vi "Main Page.vi"(8 "error in (no error)":errorcluster, 11 "Node Ptr":T3 format="%.0x") -> (0 "error out":errorcluster)   [LabVIEW 2018, in "CAN Gateway System Explorer.lvlib"]
uses:
  CAN Gateway System Explorer.lvlib
  <vilib>/NI Veristand/Custom Device API/Custom Device Item Ref.ctl
  Types/Baudrate Network Port.ctl
  Types/Baudrate DUT Port.ctl
  Types/BR Cluster.ctl
  Shared/Constants.vi
  <vilib>/NI Veristand/Custom Device API/Get Item Property (String).vi
  <vilib>/NI Veristand/Custom Device API/Set Item Property (String).vi
  <vilib>/NI Veristand/Custom Device API/Set Item Property (Variant).vi
  <vilib>/NI Veristand/Custom Device API/Custom Device API.lvlib
  Shared/CAN Gateway Shared.lvlib
panel:
  in  "CLUSTER":u16(ring)
  in  "Baudrate DUT Port":T1 items=["1 M", "500k", "250 k", "125 k", "50k"]
  in  "Baudrate Network Port":T2 items=["1 M", "500k", "250 k", "125 k", "50k"]
  out "NETWORK --> DUT Frames":string[][](table)
  out "DUT --> NETWORK Frames":string[][](table)
  in  "DUT PORT":u16(ring)
  in  "ECU":u16(ring)
  in  "NETWORK PORT":u16(ring)
  out "Database Path":string
  in  "Header":cluster{"Section Name":string}={"Section Name"="CAN Gateway Custom Device"}
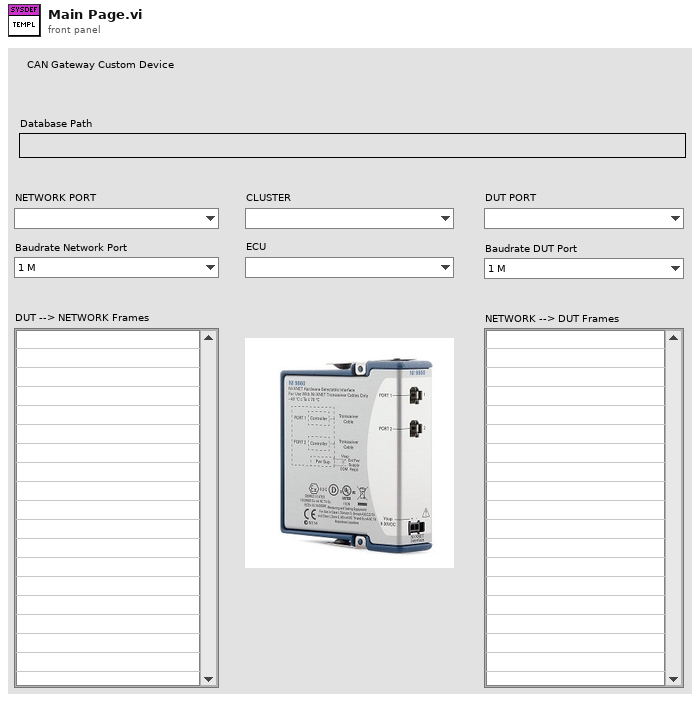
[diagram p1: front panel]
types:
  T1 = typedef "CAN Gateway System Explorer.lvlib/Baudrate DUT Port.ctl" = u16
  T2 = typedef "CAN Gateway System Explorer.lvlib/Baudrate Network Port.ctl" = u16
  T3 = typedef "Custom Device API.lvlib/Custom Device Item Ref.ctl" = u64
  T4 = typedef "CAN Gateway System Explorer.lvlib/BR Cluster.ctl" = cluster{"BR Network-Port":u16, "BR Port Network":u16}
  T5 = typedef "Custom Device API.lvlib/Custom Device Commands.ctl" = enum16{"Default", "Item renamed", "Shutdown", "Dynamic button pressed"}
  T6 = typedef "Custom Device API.lvlib/Custom Device Item Info.ctl" = cluster{"Name":string, "Is Channel":bool, "GUID":string, "Is Waveform":bool}
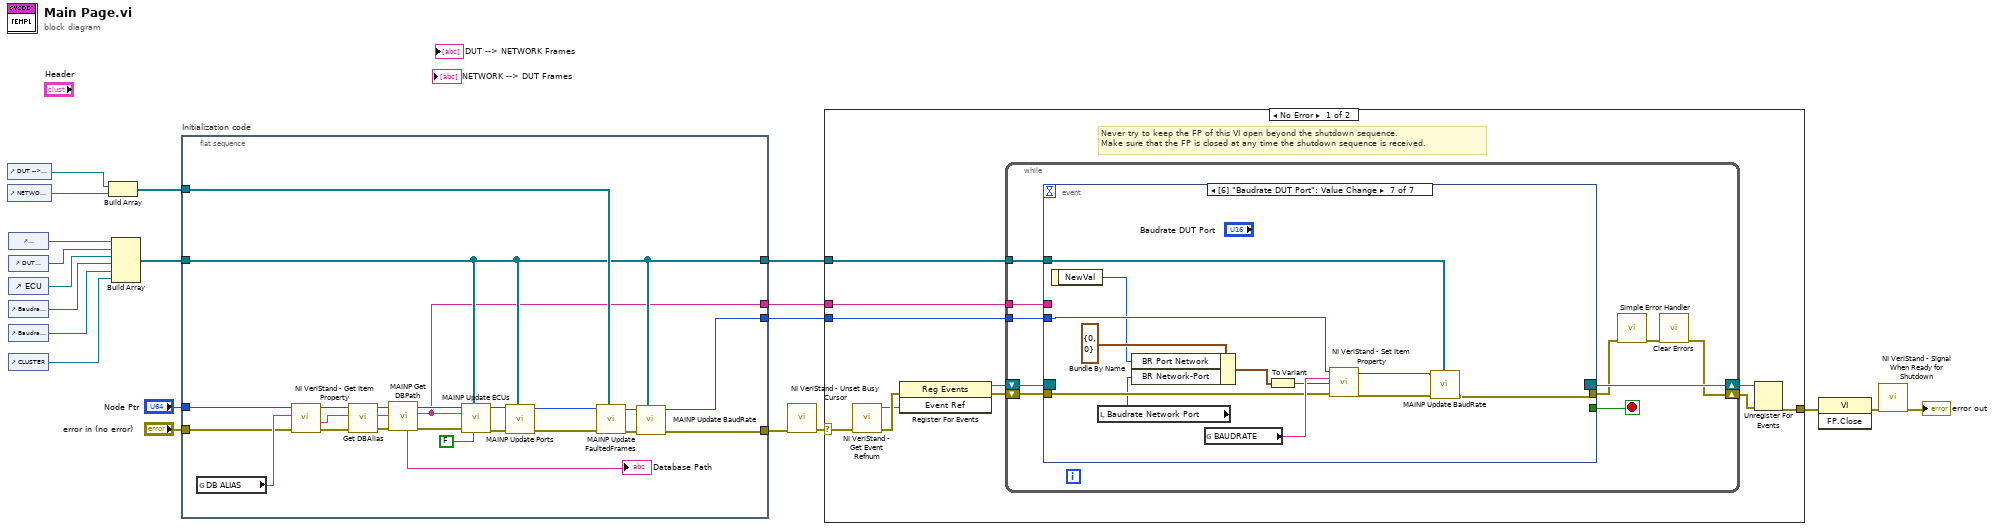
[diagram p0: block diagram]
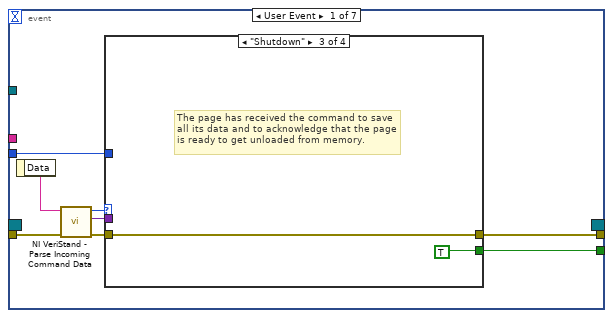
[diagram p2: hidden frame]
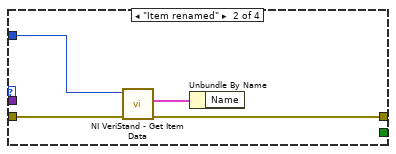
[diagram p4: hidden frame]
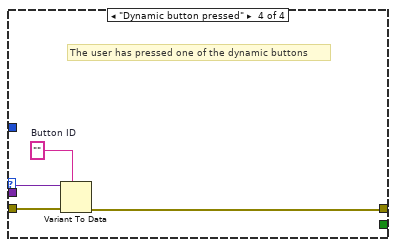
[diagram p5: hidden frame]
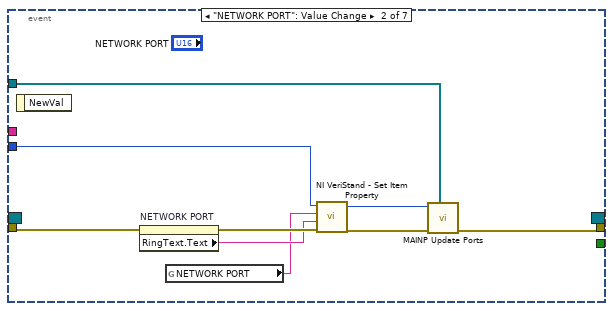
[diagram p6: hidden frame]
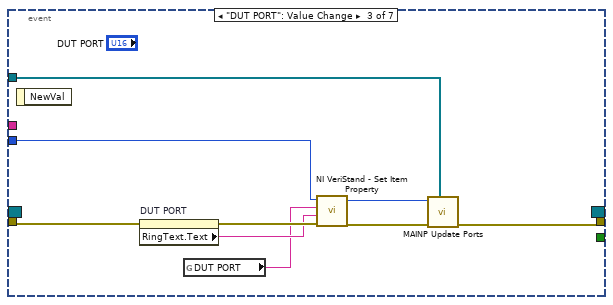
[diagram p7: hidden frame]
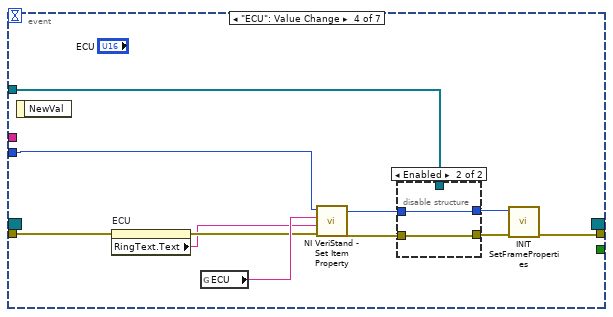
[diagram p8: hidden frame]
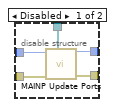
[diagram p9: hidden frame]
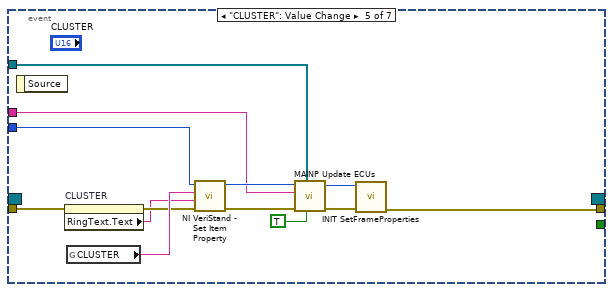
[diagram p10: hidden frame]
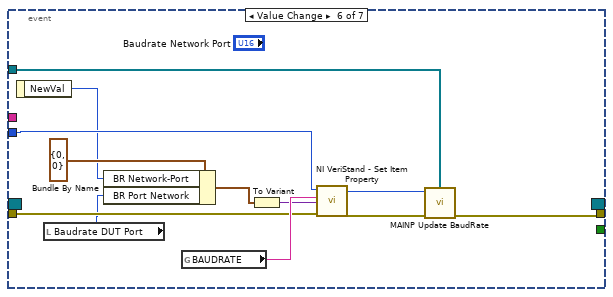
[diagram p11: hidden frame]
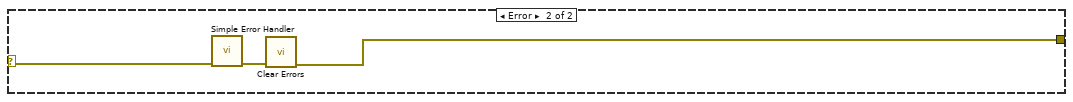
[diagram p12: hidden frame]
diagram:
  n1 = control-ref of="DUT --> NETWORK Frames"() -> (w6:refnum<vi>)
  n2 = control-ref of="NETWORK --> DUT Frames"() -> (w5:refnum<vi>)
  n3 = control-ref of="NETWORK PORT"() -> (w14:refnum<vi>)
  n4 = control-ref of="DUT PORT"() -> (w13:refnum<vi>)
  n5 = control-ref of="ECU"() -> (w10:refnum<vi>)
  n6 = control-ref of="Baudrate Network Port"() -> (w4:refnum<vi>)
  n7 = control-ref of="Baudrate DUT Port"() -> (w3:refnum<vi>)
  n8 = control-ref of="CLUSTER"() -> (w2:refnum<vi>)
  n9 = Build Array(w6, w5) -> (w7:refnum<vi>[])
  n10 = Build Array(w14, w13, w10, w4, w3, w2) -> (w12:refnum<vi>[])
  n11 = flat-sequence "Initialization code" {
    tunnel: "error in (no error)" -> [w21]
    tunnel: "Node Ptr" -> [w23]
    tunnel: w12 -> [w32]
    tunnel: [w32] -> w11
    tunnel: [w31] -> w9
    tunnel: [w33] -> w8
    tunnel: w7 -> [w36]
    tunnel: [w30] -> w1
    frame #0 {
      n12 = global read "Constants.vi" "DB ALIAS"() -> (w24:string)
      n13 = call-poly <vilib>:"NI VeriStand - Get Item Property.vi"("error in (no error)"=w21, "Property Name"=w24, "Item Ref in"=w23) -> ("error out"=w25:errorcluster, "Value"=w26:string, "Item Ref out"=w22:T3)  [unwired: 5 in, 1 out]
      n14 = call "Get DBAlias.vi"("error in (no error)"=w25, "DB Alias"=w26, "Device Item Ref in"=w22) -> ("error out"=w43:errorcluster, "Alias"=w41:string, "Device Item Ref out"=w44:T3)  [unwired: 6 in]
      n15 = call "MAINP Get DBPath.vi"("error in (no error)"=w43, "Alias"=w41, "Device Item Ref in"=w44) -> ("error out"=w39:errorcluster, "Alias"=w30:string, "Device Item Ref out"=w40:T3, "Path"=→"Database Path":string)  [unwired: 5 in]
      n16 = call "MAINP Update ECUs.vi"("First?"=FALSE, "Controls"=w32, "error in (no error)"=w39, "Alias"=w30, "Device Item Ref in"=w40) -> ("error out"=w37:errorcluster, "Device Item Ref out"=w38:T3)  [unwired: 5 in]
      n17 = call "MAINP Update Ports.vi"("Controls"=w32, "error in (no error)"=w37, "Device Item Ref in"=w38) -> ("error out"=w28:errorcluster, "Device Item Ref out"=w27:T3)  [unwired: 7 in]
      n18 = call "MAINP Update FaultedFrames.vi"("Controls"=w36, "error in (no error)"=w28, "Device Item Ref in"=w27) -> ("error out"=w35:errorcluster, "Device Item Ref out"=w34:T3)  [unwired: 7 in]
      n19 = call "MAINP Update BaudRate.vi"("Controls"=w32, "error in (no error)"=w35, "Device Item Ref in"=w34) -> ("error out"=w31:errorcluster, "Device Item Ref out"=w33:T3)  [unwired: 7 in]
    }
  }
  n20 = call <vilib>:"NI VeriStand - Unset Busy Cursor.vi"("error in (no error)"=w9) -> ("error out"=w16:errorcluster)  [unwired: 10 out]
  n21 = case shown="No Error" w16 {
    selector: w16 -> [w48 w160]
    tunnel: [w52 w158] -> w20
    tunnel: w11 -> [w47 _]
    tunnel: w8 -> [w46 _]
    tunnel: w1 -> [w45 _]
    frame No Error {
      # "Never try to keep the FP of this VI open beyond the shutdown sequence.\nMake sure that the FP is closed at any time the shutdown sequence is received."
      n22 = call <vilib>:"NI VeriStand - Get Event Refnum.vi"("error in (no error)"=w48) -> ("error out"=w55:errorcluster, "Event Ref"=w51:refnum<user-event>)  [unwired: 9 out]
      n23 = register-events(error in=w55, w51) -> (reference out=w49:refnum<event-registration>, error out=w50:errorcluster)  [unwired: 1 in]
      n24 = while {
        shift-right: [w59] -> w53
        shift-left: w50 -> [w64]
        shift-right: [w65] -> w54
        shift-left: w49 -> [w63]
        tunnel: w47 -> [w58]
        tunnel: w46 -> [w57]
        tunnel: w45 -> [w56]
        stop <- w62 stop-if-true
        n25 = event shown="[6] \"Baudrate DUT Port\": Value Change" {
          selector: w63 -> [_ _ _ _ _ _ _]
          dyn-events: [_ _ _ _ _ _ _] -> w65
          timeout: _ -> [_ _ _ _ _ _ _]
          tunnel: w64 -> [w73 w93 w102 w108 w131 w142 w154]
          tunnel: [w69 _ _ _ _ _ _] -> w62
          tunnel: [w68 w87 w96 w103 w121 w135 w147] -> w61
          tunnel: w58 -> [_ w86 w95 w110 w128 w136 w148]
          tunnel: w57 -> [w66 w85 w94 w106 w132 w144 w156]
          tunnel: w56 -> [_ _ _ _ w125 _ _]
          event User Event {
            n26 = event-data() -> ("Data"=w72:string)  [unwired: 1 out]
            n27 = call <vilib>:"NI VeriStand - Parse Incoming Command Data.vi"("error in (no error)"=w73, "Incoming data"=w72) -> ("error out"=w71:errorcluster, "Outgoing data"=w67:variant, "Action"=w70:T5)  [unwired: 7 out]
            n28 = case shown="\"Shutdown\"" w70 {
              tunnel: w71 -> [w74 w78 w79 w84]
              tunnel: [_ _ TRUE _] -> w69
              tunnel: [w74 w76 w79 w81] -> w68
              tunnel: w67 -> [_ _ _ w83]
              tunnel: w66 -> [_ w75 _ _]
              frame "Default", Default {
              }
              frame "Item renamed" {
                n29 = call <vilib>:"NI VeriStand - Get Item Data.vi"("error in (no error)"=w78, "Item Ref in"=w75) -> ("error out"=w76:errorcluster, "Item Info"=w77:T6)  [unwired: 8 out]
                n30 = Unbundle By Name(w77) -> ()  [unwired: 1 out]
              }
              frame "Shutdown" {
                # "The page has received the command to save all its data and to acknowledge that the page is ready to get unloaded from memory."
              }
              frame "Dynamic button pressed" {
                w82 = ""  # Button ID
                # "The user has pressed one of the dynamic buttons"
                n31 = Variant To Data(error in=w84, type=w82, Variant=w83) -> (error out=w81:errorcluster)  [unwired: 1 out]
              }
            }
          }
          event "NETWORK PORT": Value Change {
            n32 = event-data() -> ()  [unwired: 2 out]
            n33 = property on="NETWORK PORT" class="Ring (strict)"(error in=w93) -> (error out=w92:errorcluster, "RingText.Text"=w91:string)  [unwired: 1 in, 1 out]
            n34 = global read "Constants.vi" "NETWORK PORT"() -> (w90:string)
            n35 = call-poly <vilib>:"NI VeriStand - Set Item Property.vi"("error in (no error)"=w92, "Value"=w91, "Property Name"=w90, "Item Ref in"=w85) -> ("error out"=w89:errorcluster, "Item Ref out"=w88:T3)  [unwired: 5 in, 1 out]
            n36 = call "MAINP Update Ports.vi"("Controls"=w86, "error in (no error)"=w89, "Device Item Ref in"=w88) -> ("error out"=w87:errorcluster)  [unwired: 7 in, 1 out]
          }
          event "DUT PORT": Value Change {
            n37 = event-data() -> ()  [unwired: 2 out]
            n38 = property on="DUT PORT" class="Ring (strict)"(error in=w102) -> (error out=w101:errorcluster, "RingText.Text"=w100:string)  [unwired: 1 in, 1 out]
            n39 = global read "Constants.vi" "DUT PORT"() -> (w99:string)
            n40 = call-poly <vilib>:"NI VeriStand - Set Item Property.vi"("error in (no error)"=w101, "Value"=w100, "Property Name"=w99, "Item Ref in"=w94) -> ("error out"=w98:errorcluster, "Item Ref out"=w97:T3)  [unwired: 5 in, 1 out]
            n41 = call "MAINP Update Ports.vi"("Controls"=w95, "error in (no error)"=w98, "Device Item Ref in"=w97) -> ("error out"=w96:errorcluster)  [unwired: 7 in, 1 out]
          }
          event "ECU": Value Change {
            n42 = event-data() -> ()  [unwired: 2 out]
            n43 = property on="ECU" class="Ring (strict)"(error in=w108) -> (error out=w109:errorcluster, "RingText.Text"=w107:string)  [unwired: 1 in, 1 out]
            n44 = global read "Constants.vi" "ECU"() -> (w113:string)
            n45 = call-poly <vilib>:"NI VeriStand - Set Item Property.vi"("error in (no error)"=w109, "Value"=w107, "Property Name"=w113, "Item Ref in"=w106) -> ("error out"=w112:errorcluster, "Item Ref out"=w111:T3)  [unwired: 5 in, 1 out]
            n46 = disable-structure shown="Enabled" {
              disable-tunnel: w112 -> [w118 w119]
              disable-tunnel: w111 -> [w117 w120]
              disable-tunnel: w110 -> [w116 _]
              disable-tunnel: [w115 w119] -> w105
              disable-tunnel: [w114 w120] -> w104
              frame Disabled {
                n47 = call "MAINP Update Ports.vi"("Controls"=w116, "error in (no error)"=w118, "Device Item Ref in"=w117) -> ("error out"=w115:errorcluster, "Device Item Ref out"=w114:T3)  [unwired: 7 in]
              }
              frame Enabled {
              }
            }
            n48 = call "INIT SetFrameProperties.vi"("error in (no error)"=w105, "Device Item Ref in"=w104) -> ("error out"=w103:errorcluster)  [unwired: 8 in, 1 out]
          }
          event "CLUSTER": Value Change {
            n49 = event-data() -> ()  [unwired: 2 out]
            n50 = property on="CLUSTER" class="Ring (strict)"(error in=w131) -> (error out=w130:errorcluster, "RingText.Text"=w129:string)  [unwired: 1 in, 1 out]
            n51 = global read "Constants.vi" "CLUSTER"() -> (w133:string)
            n52 = call-poly <vilib>:"NI VeriStand - Set Item Property.vi"("error in (no error)"=w130, "Value"=w129, "Property Name"=w133, "Item Ref in"=w132) -> ("error out"=w127:errorcluster, "Item Ref out"=w126:T3)  [unwired: 5 in, 1 out]
            n53 = call "MAINP Update ECUs.vi"("First?"=TRUE, "Controls"=w128, "error in (no error)"=w127, "Alias"=w125, "Device Item Ref in"=w126) -> ("error out"=w124:errorcluster, "Device Item Ref out"=w123:T3)  [unwired: 5 in]
            n54 = call "INIT SetFrameProperties.vi"("error in (no error)"=w124, "Device Item Ref in"=w123) -> ("error out"=w121:errorcluster)  [unwired: 8 in, 1 out]
          }
          event Value Change {
            n55 = event-data() -> ("NewVal"=w139:T2)  [unwired: 1 out]
            n56 = local read "Baudrate DUT Port"() -> (w134:T1)
            n57 = Bundle By Name(cluster=T4 {"BR Network-Port"=0, "BR Port Network"=0} ("BR Cluster"), "BR Network-Port"=w139, "BR Port Network"=w134) -> (w140:T4)
            n58 = global read "Constants.vi" "BAUDRATE"() -> (w145:string)
            n59 = To Variant(anything=w140) -> (Variant=w141:variant)
            n60 = call-poly <vilib>:"NI VeriStand - Set Item Property.vi"("error in (no error)"=w142, "Value"=w141, "Property Name"=w145, "Item Ref in"=w144) -> ("error out"=w137:errorcluster, "Item Ref out"=w138:T3)  [unwired: 5 in, 1 out]
            n61 = call "MAINP Update BaudRate.vi"("Controls"=w136, "error in (no error)"=w137, "Device Item Ref in"=w138) -> ("error out"=w135:errorcluster)  [unwired: 7 in, 1 out]
          }
          event Value Change {
            n62 = event-data() -> ("NewVal"=w151:T1)  [unwired: 1 out]
            n63 = local read "Baudrate Network Port"() -> (w146:T2)
            n64 = Bundle By Name(cluster=T4 {"BR Network-Port"=0, "BR Port Network"=0} ("BR Cluster"), "BR Port Network"=w151, "BR Network-Port"=w146) -> (w152:T4)
            n65 = global read "Constants.vi" "BAUDRATE"() -> (w157:string)
            n66 = To Variant(anything=w152) -> (Variant=w153:variant)
            n67 = call-poly <vilib>:"NI VeriStand - Set Item Property.vi"("error in (no error)"=w154, "Value"=w153, "Property Name"=w157, "Item Ref in"=w156) -> ("error out"=w150:errorcluster, "Item Ref out"=w149:T3)  [unwired: 5 in, 1 out]
            n68 = call "MAINP Update BaudRate.vi"("Controls"=w148, "error in (no error)"=w150, "Device Item Ref in"=w149) -> ("error out"=w147:errorcluster)  [unwired: 7 in, 1 out]
          }
        }
        n69 = call <vilib>:"Simple Error Handler.vi"("error in (no error)"=w61) -> ("error out"=w60:errorcluster)  [unwired: 1 in, 7 out]
        n70 = call <vilib>:"Clear Errors.vi"("error in (no error)"=w60) -> ("error out"=w59:errorcluster)  [unwired: 1 in, 5 out]
      }
      n71 = Unregister For Events(event registration refnum=w54, error in=w53) -> (error out=w52:errorcluster)
    }
    frame Error {
      n72 = call <vilib>:"Simple Error Handler.vi"("error in (no error)"=w160) -> ("error out"=w159:errorcluster)  [unwired: 1 in, 7 out]
      n73 = call <vilib>:"Clear Errors.vi"("error in (no error)"=w159) -> ("error out"=w158:errorcluster)  [unwired: 1 in, 5 out]
    }
  }
  n74 = invoke class="VI" method="FP.Close"(error in=w20) -> (error out=w19:errorcluster)  [unwired: 2 in, 2 out]
  n75 = call <vilib>:"NI VeriStand - Signal When Ready for Shutdown.vi"("error in (no error)"=w19) -> ("error out"=→"error out":errorcluster)  [unwired: 10 out]
